vi "Tosca-Send AI Command.vi"(0 "action":string, 7 "Variant":variant, 11 "error in (no error)":errorcluster) -> (15 "error out":errorcluster)   [LabVIEW 2020]
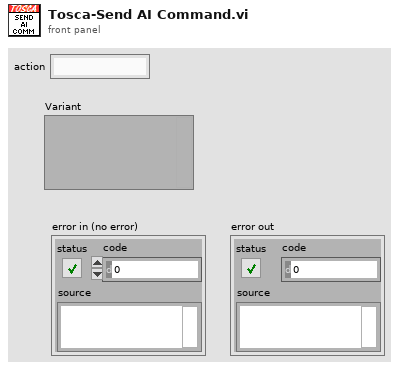
[diagram p1: front panel]
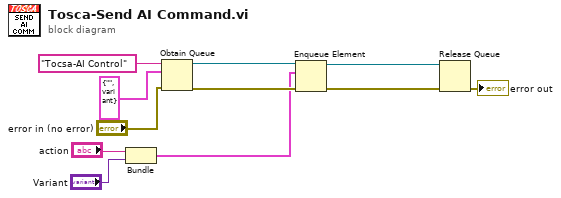
[diagram p0: block diagram]
diagram:
  n1 = Bundle("action"="action", "Variant"="Variant") -> (w5:cluster{"action":string, "Variant":variant})  [unwired: 1 in]
  n2 = Obtain Queue(name (unnamed)="Tocsa-AI Control", element data type=cluster{"Action":string, "Data":variant} {"Action"="", "Data"=variant} ("Data"), error in (no error)="error in (no error)") -> (queue out=w6:refnum<queue>, error out=w7:errorcluster)  [unwired: 2 in, 1 out]
  n3 = Enqueue Element(queue=w6, element=w5, error in (no error)=w7) -> (queue out=w3:refnum<queue>, error out=w2:errorcluster)  [unwired: 1 in, 1 out]
  n4 = Release Queue(queue=w3, error in (no error)=w2) -> (error out=→"error out":errorcluster)  [unwired: 1 in, 2 out]
